vi "SimulatorLoop updated.vi"() -> ()   [LabVIEW 2016]
uses:
  Z:/LiSARD_Reference_Project/Multicore_1.6beta/CodeConverter/Controls/EX.Command.ctl
  Z:/LiSARD_Reference_Project/Multicore_1.6beta/CodeConverter/SoftCoreCodeConverter.lvlib
  Z:/LiSARD_Reference_Project/Multicore_1.6beta/CodeConverter/Controls/WB.Operation.ctl
  Z:/LiSARD_Reference_Project/Multicore_1.6beta/CodeConverter/Controls/CommandLine.ctl
panel:
  in  "CoreCode":T1[][](array[typedef])
  out "output array":u64[](array[numeric])
  out "element 2":u64
  out "element":u64
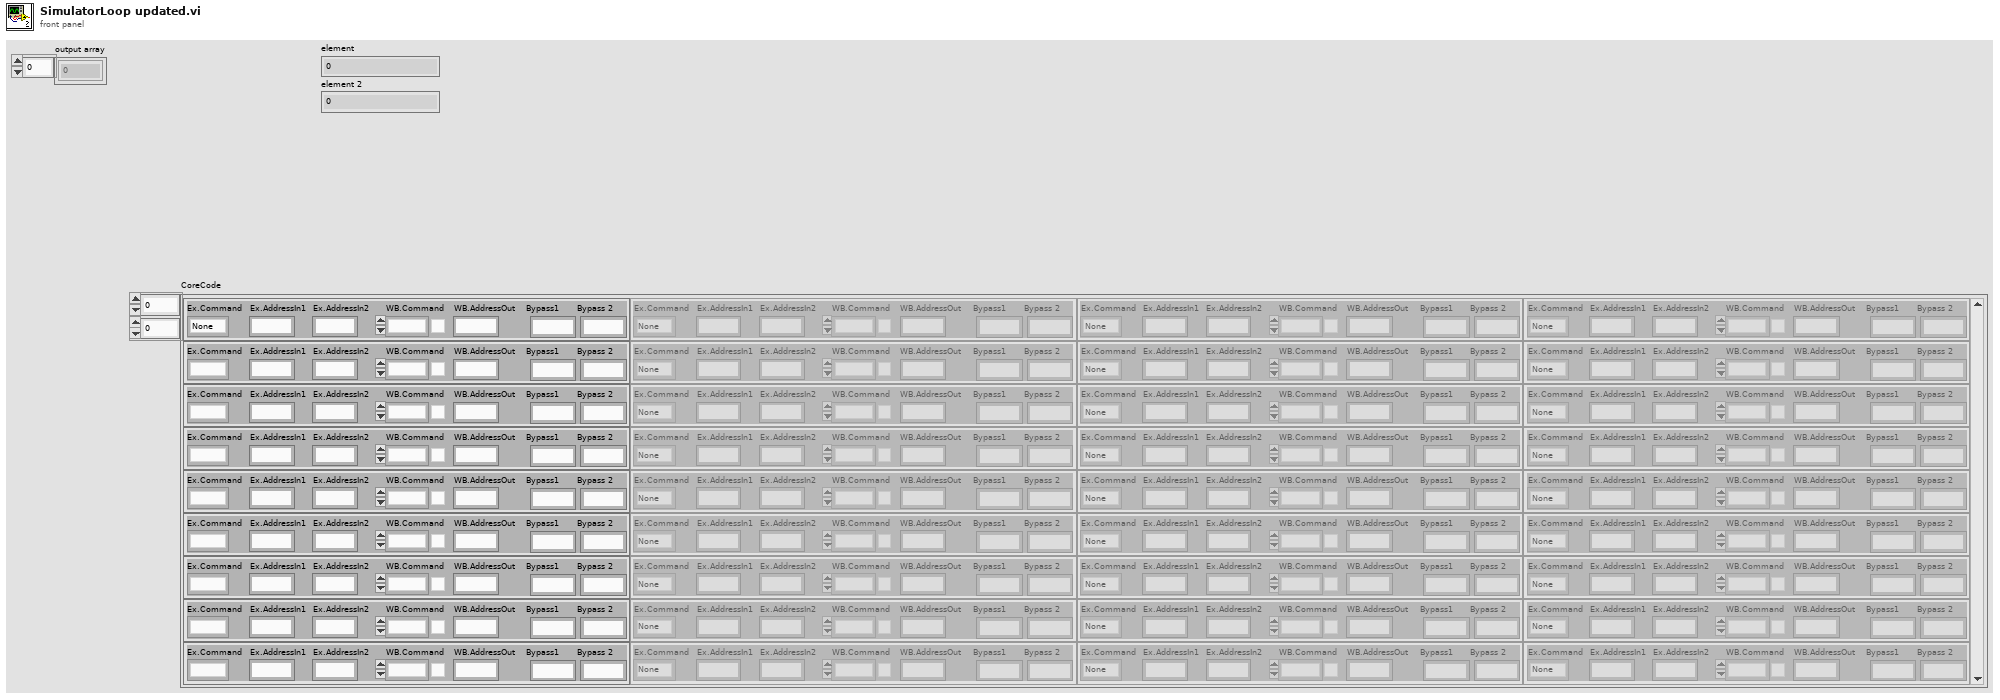
[diagram p1: front panel]
types:
  T1 = typedef "SoftCoreCodeConverter.lvlib/CommandLine.ctl" = cluster{"Ex.Command":T2, "Ex.AddressIn1":fxp<+,16,16>, "Ex.AddressIn2":fxp<+,16,16>, "WB.Command":T3, "WB.AddressOut":fxp<+,16,16>, "Bypass1":fxp<+,2,2>, "Bypass 2":fxp<+,2,2>}
  T2 = typedef "SoftCoreCodeConverter.lvlib/EX.Command.ctl" = enum8{"Default", "Sub", "None", "Fuse", "Abs", "AbsSub", "Const"}
  T3 = typedef "SoftCoreCodeConverter.lvlib/WB.Operation.ctl" = enum8{"In", "Out", "Mov", "Add", "Sub", "Mul", "Div", "None", "Sqr", "Sin", "Cos", "Sgl2Dbl", "Dbl2Int", "Int2Dbl", "Mlookup", "Dbl2Sgl", "G_IsPOS", "G_IsNEG", "G_IsNULL", "G_IsNNULL", "G_IsNAN", "G_IsNNAN", "G_IsIFTY", "G_IsNIFTY", "reserved_0", "reserved_1", "reserved_2", "reserved_3", "reserved_4", "reserved_5", "reserved_6", "reserved_7"}
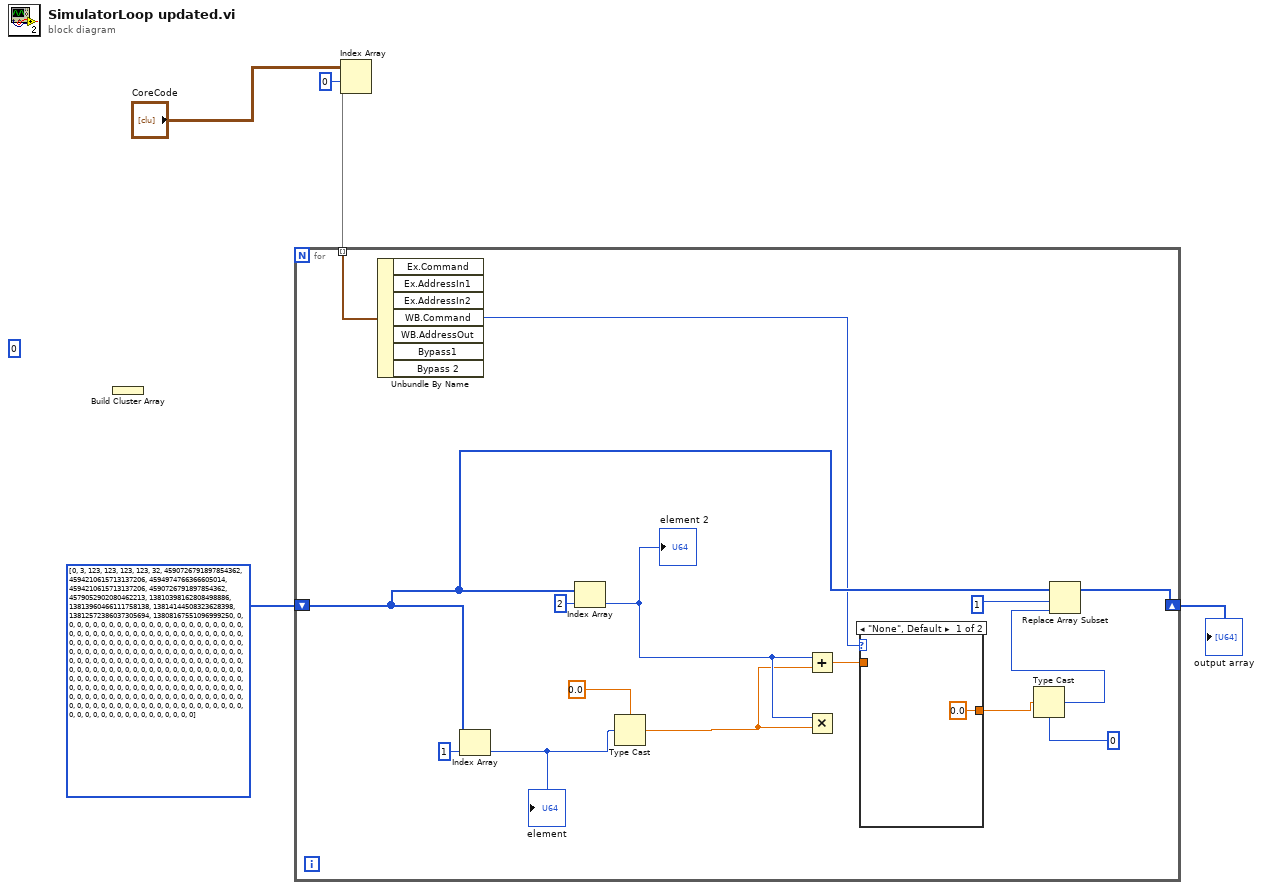
[diagram p0: block diagram]
diagram:
  (unwired) 0
  n1 = Build Cluster Array() -> ()  [unwired: 1 in, 1 out]
  n2 = Index Array(array="CoreCode", index (row)=0) -> (element=w1:T1[])  [unwired: 1 in]
  n3 = for {
    shift-right: [w16] -> w4
    shift-left: u64[] [0, 3, 123, 123, 123, 123, 32, 4590726791897854362, 4594210615713137206, 4594974766366605014, 4594210615713137206, 4590726791897854362, 4579052902080462213, 13810398162808498886, 13813960466111758138, 13814144508323628398, 13812572386037305694, 13808167551096999250, 0, 0, 0, 0, 0, 0, 0, 0, 0, 0, 0, 0, 0, 0, 0, 0, 0, 0, 0, 0, 0, 0, 0, 0, 0, 0, 0, 0, 0, 0, 0, 0, 0, 0, 0, 0, 0, 0, 0, 0, 0, 0, 0, 0, 0, 0, 0, 0, 0, 0, 0, 0, 0, 0, 0, 0, 0, 0, 0, 0, 0, 0, 0, 0, 0, 0, 0, 0, 0, 0, 0, 0, 0, 0, 0, 0, 0, 0, 0, 0, 0, 0, 0, 0, 0, 0, 0, 0, 0, 0, 0, 0, 0, 0, 0, 0, 0, 0, 0, 0, 0, 0, 0, 0, 0, 0, 0, 0, 0, 0, 0, 0, 0, 0, 0, 0, 0, 0, 0, 0, 0, 0, 0, 0, 0, 0, 0, 0, 0, 0, 0, 0, 0, 0, 0, 0, 0, 0, 0, 0, 0, 0, 0, 0, 0, 0, 0, 0, 0, 0, 0, 0, 0, 0, 0, 0, 0, 0, 0, 0, 0, 0, 0, 0, 0, 0, 0, 0, 0, 0, 0, 0, 0, 0, 0, 0, 0, 0, 0, 0, 0, 0, 0, 0, 0, 0, 0, 0, 0, 0, 0, 0, 0, 0, 0, 0, 0, 0, 0, 0, 0, 0, 0, 0, 0, 0, 0, 0, 0, 0, 0, 0, 0, 0, 0, 0, 0, 0, 0, 0, 0, 0, 0, 0, 0, 0, 0, 0, 0, 0, 0, 0, 0, 0, 0, 0, 0] ("DataMemory/Fxp") -> [w20]
    tunnel: w1 -> [w15] mode=indexing
    n4 = Unbundle By Name(w15) -> ("WB.Command"=w13:T3)  [unwired: 6 out]
    n5 = Index Array "Index Array"(array=w20, index=1) -> (element=w11:u64)
    "element" <- w11
    n6 = Index Array "Index Array"(array=w20, index=2) -> (element=w14:u64)
    "element 2" <- w14
    n7 = Type Cast(type=0.0, x=w11) -> (*(type *) &x=w9:dbl)
    n8 = Add(x=w14, y=w9) -> (x+y=w12:dbl)
    n9 = Multiply(x=w14, y=w9) -> ()  [unwired: 1 out]
    n10 = case shown="\"None\", Default" w13 {
      tunnel: [0.0 w22] -> w7
      tunnel: w12 -> [_ w22]
      frame "None", Default {
      }
      frame "Add" {
      }
    }
    n11 = Type Cast(type=u64 0, x=w7) -> (*(type *) &x=w6:u64)
    n12 = Replace Array Subset "Replace Array Subset"(array=w20, new element=w6, index=1) -> (w16:u64[])
  }
  "output array" <- w4
